vi "Read User Tag.vi"(8 "error in (no error)":errorcluster, 11 "NT Base in":refnum<class "NT Base.lvclass">) -> (0 "error out":errorcluster, 2 "user tag":i32, 3 "NT Base out":refnum<class "NT Base.lvclass">)   [LabVIEW 2020, in "PV Access.lvlib" / "PV Data.lvlib" / "NT Base.lvclass"]
uses:
  NT Base.lvclass
  NT Base.lvclass/NT Base.ctl
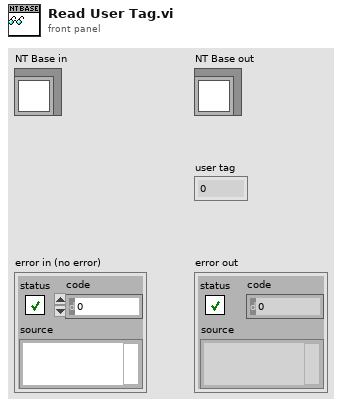
[diagram p1: front panel]
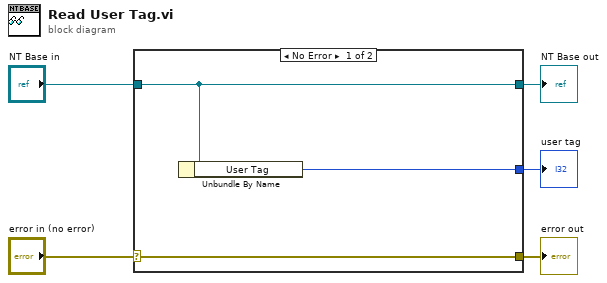
[diagram p0: block diagram]
diagram:
  n1 = case shown="No Error" "error in (no error)" {
    selector: "error in (no error)" -> [w8 w9]
    tunnel: [w8 w9] -> w4
    tunnel: [w7 w10] -> w2
    tunnel: "NT Base in" -> [w7 w10]
    tunnel: [w6 _] -> w1
    frame No Error {
      n2 = Unbundle By Name(w7) -> ("User Tag"=w6:i32)
    }
    frame Error {
    }
  }
  "error out" <- w4
  "NT Base out" <- w2
  "user tag" <- w1
